vi "Global_Autonomous_Route.vi"() -> ()   [LabVIEW 2017]
uses:
  Systems/Autonomous/Autonomous/ENUM_Auto_AutoMode.ctl
panel:
  in  "Auto Route":T1
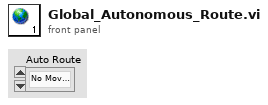
[diagram p1: front panel]
types:
  T1 = typedef "ENUM_Auto_AutoMode.ctl" = enum16{"No Movement", "Scale And Switch", "Switch", "Scale", "Cross Line"}
diagram:
